vi "Staib EG.vi"(0 "QUIT":refnum<vi>, 1 "Scan in Progress":refnum<vi>, 2 "Set EG":refnum<vi>, 3 "Energy (eV)":refnum<vi>, 4 "Extraction (V)":refnum<vi>, 5 "Filament (V)":refnum<vi>, 6 "EG Computer Control":refnum<vi>, 7 "X1 Alignment (V)":refnum<vi>, 8 "Error":refnum<vi>, 9 "X2 Alignment (V)":refnum<vi>, 11 "Y1 Alignment (V)":refnum<vi>, 13 "Y2 Alignment (V)":refnum<vi>, 14 "Grid (V)":refnum<vi>, 15 "Focus 1 (V)":refnum<vi>, 16 "Focus 2 (V)":refnum<vi>) -> ()   [LabVIEW 2018]
uses:
  <vilib>/DAQmx/write.llb/DAQmx Write (Analog DBL 1Chan 1Samp).vi
  <vilib>/DAQmx/write.llb/DAQmx Write (Digital Bool 1Line 1Point).vi
panel:
  in  "Staib Electron Gun":enum32{"Controls", "Settings"}(tab)
  in  "Lock Focus Knobs":bool
  out "Computer\nControl Enabled?":bool
  in  "Computer\nControl":bool
  in  "Y2 Alignment (V)":dbl(knob) min=-10.0 max=10.0 step=0.001 scale=-10.0..10.0 scale format="%#_3g"
  in  "Y1 Alignment (V)":dbl(knob) min=-10.0 max=10.0 step=0.001 scale=-10.0..10.0 scale format="%#_3g"
  in  "X2 Alignment (V)":dbl(knob) min=-10.0 max=10.0 step=0.001 scale=-10.0..10.0 scale format="%#_3g"
  in  "X1 Alignment (V)":dbl(knob) min=-10.0 max=10.0 step=0.001 scale=-10.0..10.0 scale format="%#_3g"
  in  "Filament (V)":dbl(knob) min=0.0 max=10.0 step=0.001 scale=0.0..5.0 scale format="%#_3g"
  in  "Focus 2 (V)":dbl(knob) min=-0.0 max=0.0 step=0.001 scale=0.0..0.001 scale format="%#_3g"
  in  "Focus 1 (V)":dbl(knob) min=-0.0 max=0.0 step=0.001 scale=0.0..0.001 scale format="%#_3g"
  in  "Extraction (V)":dbl(knob) min=0.0 max=100.0 step=0.001 scale=0.0..100.0 scale format="%#_3g"
  in  "Energy (eV)":dbl(knob) min=0.0 max=100.0 step=0.001 scale=0.0..100.0 scale format="%#_3g"
  in  "Grid (V)":dbl(knob) min=-15.0 max=15.0 step=0.001 scale=-15.0..15.0 scale format="%#_3g"
  out "Feedback Extraction":dbl caption="Ext"
  out "Feedback Filament":dbl caption="Fil"
  out "Feedback Energy":dbl caption="En"
  out "Feedback Grid":dbl caption="G"
  out "Feedback Focus 1":dbl caption="F 1"
  out "Feedback Focus 2":dbl caption="F 2"
  out "Feedback X1 Alignment":dbl caption="X1"
  out "Feedback X2 Alignment":dbl caption="X2"
  out "Feedback Y1 Alignment":dbl caption="Y1"
  out "Feedback Y2 Alignment":dbl caption="Y2"
  out "Focus Max (V)":dbl min=0.0 max=100.0 step=0.001
  out "Focus Min (V)":dbl
  out "Focus Disable":i32
  in  "Minimum Upper Limit of Focus' Scale (V)":dbl=0.001 min=1e-05 max=100.0 step=0.001
  # "Note that there is no feedback from the electron gun's hardware.  Check the controller's LEDs if unsure."
  # "On"
  # "Off"
  # "Software Feedback"
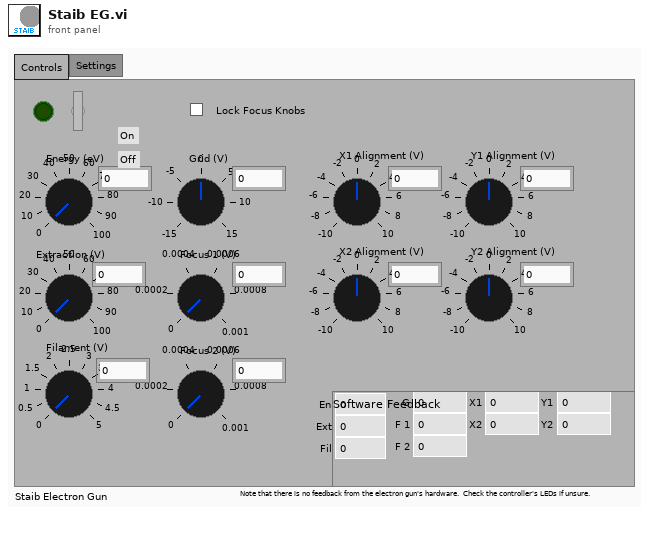
[diagram p1: front panel]
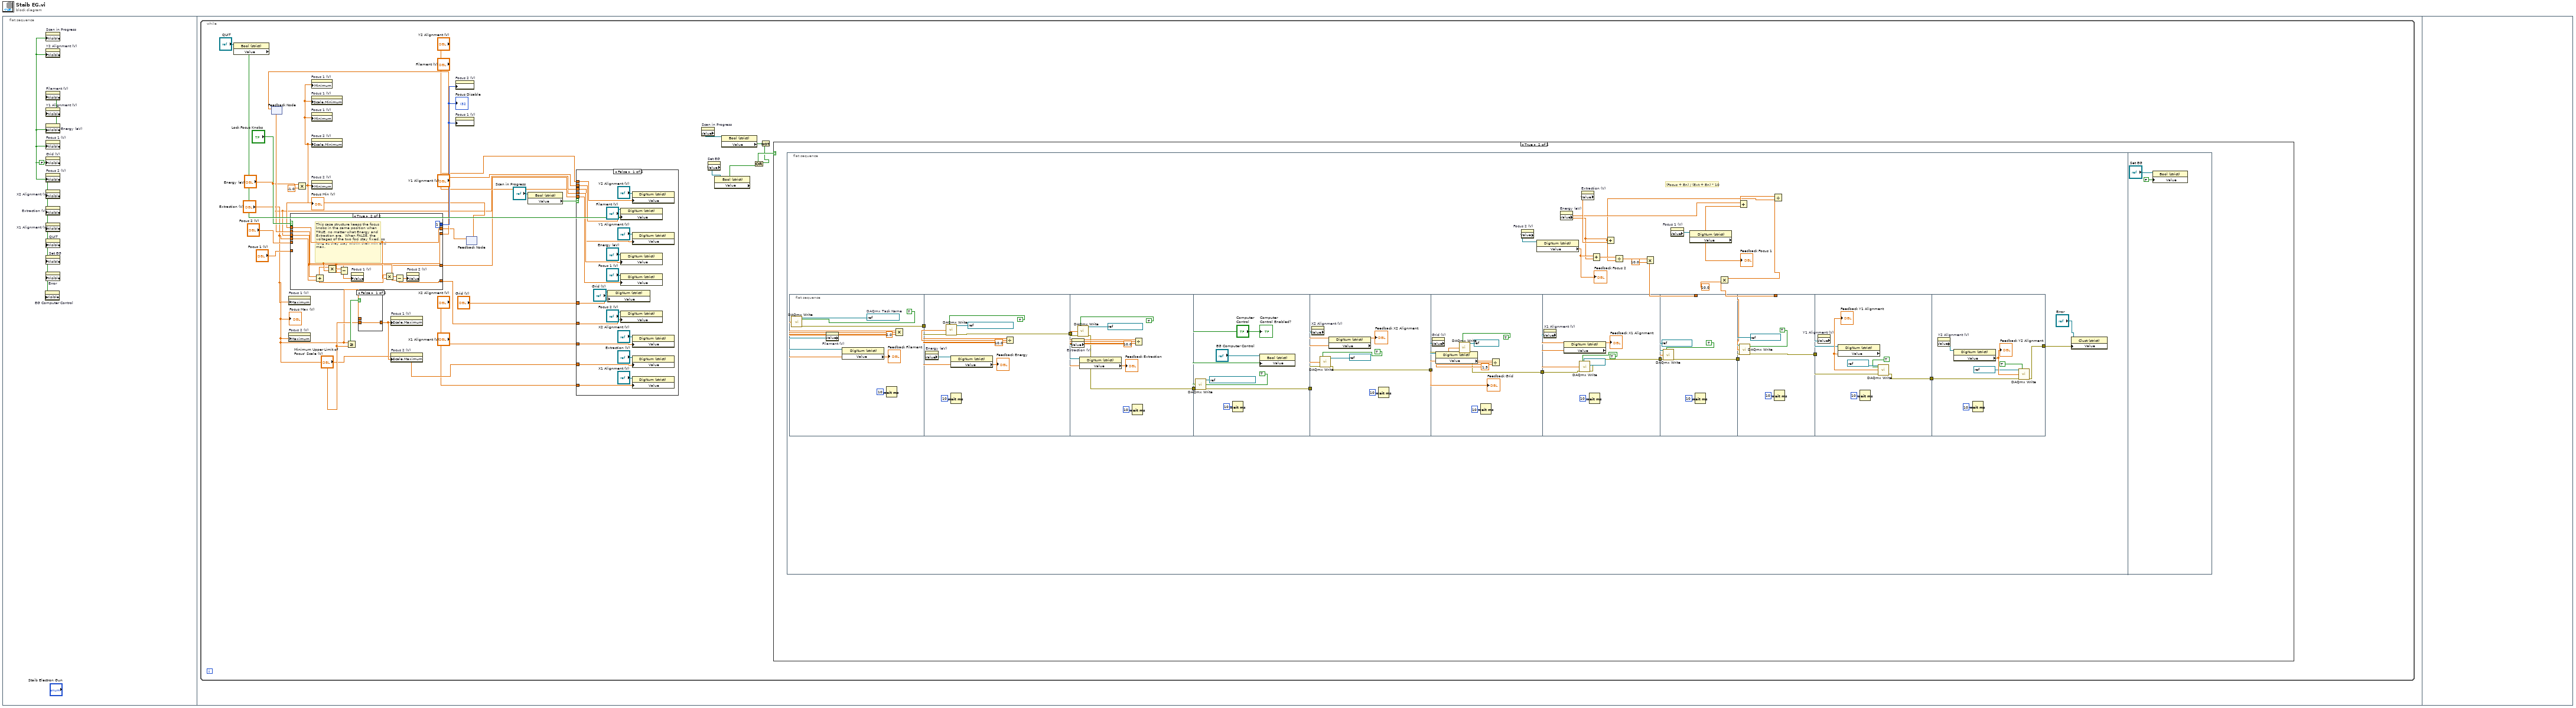
[diagram p0: block diagram]
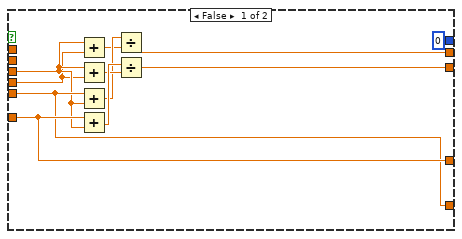
[diagram p5: hidden frame]
diagram:
  n1 = flat-sequence {
    frame #0 {
      w1 = FALSE ("Visible")
      n2 = property on="EG Computer Control" class="LVObjRef (strict)"("Visible"=w1) -> ()  [unwired: 2 in, 2 out]
      n3 = property on="Scan in Progress" class="LVObjRef (strict)"("Visible"=w1) -> ()  [unwired: 2 in, 2 out]
      n4 = property on="Y2 Alignment (V)" class="LVObjRef (strict)"("Visible"=w1) -> ()  [unwired: 2 in, 2 out]
      n5 = property on="Filament (V)" class="LVObjRef (strict)"("Visible"=w1) -> ()  [unwired: 2 in, 2 out]
      n6 = property on="Y1 Alignment (V)" class="LVObjRef (strict)"("Visible"=w1) -> ()  [unwired: 2 in, 2 out]
      n7 = property on="Energy (eV)" class="LVObjRef (strict)"("Visible"=w1) -> ()  [unwired: 2 in, 2 out]
      n8 = property on="Focus 1 (V)" class="LVObjRef (strict)"("Visible"=w1) -> ()  [unwired: 2 in, 2 out]
      n9 = property on="Grid (V)" class="LVObjRef (strict)"("Visible"=w1) -> ()  [unwired: 2 in, 2 out]
      n10 = property on="Focus 2 (V)" class="LVObjRef (strict)"("Visible"=w1) -> ()  [unwired: 2 in, 2 out]
      n11 = property on="X2 Alignment (V)" class="LVObjRef (strict)"("Visible"=w1) -> ()  [unwired: 2 in, 2 out]
      n12 = property on="Extraction (V)" class="LVObjRef (strict)"("Visible"=w1) -> ()  [unwired: 2 in, 2 out]
      n13 = property on="X1 Alignment (V)" class="LVObjRef (strict)"("Visible"=w1) -> ()  [unwired: 2 in, 2 out]
      n14 = property on="QUIT" class="LVObjRef (strict)"("Visible"=w1) -> ()  [unwired: 2 in, 2 out]
      n15 = property on="Set EG" class="LVObjRef (strict)"("Visible"=w1) -> ()  [unwired: 2 in, 2 out]
      n16 = property on="Error" class="LVObjRef (strict)"("Visible"=w1) -> ()  [unwired: 2 in, 2 out]
    }
    frame #1 {
      n17 = while {
        stop <- w33 stop-if-true
        n18 = property class="Bool (strict)"(reference="QUIT") -> ("Value"=w33:bool)  [unwired: 1 in, 2 out]
        n19 = feedback #1() -> (w26:dbl)  [unwired: 1 in]
        n20 = property on="Focus 1 (V)" class="Knob (strict)"("Maximum"="Extraction (V)") -> ()  [unwired: 2 in, 2 out]
        n21 = property on="Focus 2 (V)" class="Knob (strict)"("Maximum"="Extraction (V)") -> ()  [unwired: 2 in, 2 out]
        n22 = Multiply(x="Energy (eV)", y=-1.0) -> (x*y=w21:dbl)
        "Focus Min (V)" <- w21
        n23 = property on="Focus 1 (V)" class="Knob (strict)"("Minimum"=w21) -> ()  [unwired: 2 in, 2 out]
        n24 = property on="Focus 1 (V)" class="Knob (strict)"("Scale.Minimum"=w21) -> ()  [unwired: 2 in, 2 out]
        n25 = property on="Focus 1 (V)" class="Knob (strict)"("Minimum"=w21) -> ()  [unwired: 2 in, 2 out]
        n26 = property on="Focus 2 (V)" class="Knob (strict)"("Scale.Minimum"=w21) -> ()  [unwired: 2 in, 2 out]
        n27 = property on="Focus 2 (V)" class="Knob (strict)"("Minimum"=w21) -> ()  [unwired: 2 in, 2 out]
        n28 = Greater Or Equal?(x="Extraction (V)", y="Minimum Upper Limit of Focus' Scale (V)") -> (x >= y?=w23:bool)
        n29 = case shown="False" w23 {
          tunnel: "Extraction (V)" -> [_ w167]
          tunnel: [w166 w167] -> w22
          tunnel: "Minimum Upper Limit of Focus' Scale (V)" -> [w166 _]
          frame False {
          }
          frame True {
          }
        }
        n30 = property on="Focus 1 (V)" class="Knob (strict)"("Scale.Maximum"=w22) -> ()  [unwired: 2 in, 2 out]
        n31 = property on="Focus 2 (V)" class="Knob (strict)"("Scale.Maximum"=w22) -> ()  [unwired: 2 in, 2 out]
        n32 = feedback #2() -> (w24:dbl)  [unwired: 1 in]
        n33 = case shown="True" "Lock Focus Knobs" {
          tunnel: "Focus 2 (V)" -> [w171 _]
          tunnel: [w171 w179] -> w15
          tunnel: "Focus 1 (V)" -> [w177 _]
          tunnel: [w177 w180] -> w16
          tunnel: [0 1] -> w30
          tunnel: "Energy (eV)" -> [w170 w181]
          tunnel: "Extraction (V)" -> [w169 w187]
          tunnel: [w174 w185] -> w27
          tunnel: [w168 w183] -> w25
          tunnel: w26 -> [_ w185]
          tunnel: w24 -> [_ w183]
          frame False {
            n34 = Add(x=w170, y=w169) -> (x+y=w172:dbl)
            n35 = Add(x=w170, y=w169) -> (x+y=w175:dbl)
            n36 = Add(x=w171, y=w170) -> (x+y=w173:dbl)
            n37 = Add(x=w177, y=w170) -> (x+y=w176:dbl)
            n38 = Divide(x=w173, y=w172) -> (x/y=w168:dbl)
            n39 = Divide(x=w176, y=w175) -> (x/y=w174:dbl)
          }
          frame True {
            # "This case structure keeps the focus knobs in the same position when TRUE, no matter what Energy and Extraction are.  When FALSE, the voltages of the two foci stay fixed, so long as they stay within their min and max."
            n40 = Add(x=w181, y=w187) -> (x+y=w184:dbl)
            n41 = Multiply(x=w184, y=w185) -> (x*y=w186:dbl)
            n42 = Subtract(x=w186, y=w181) -> (x-y=w180:dbl)
            n43 = property on="Focus 1 (V)" class="Knob (strict)"("Value"=w180) -> ()  [unwired: 2 in, 2 out]
            n44 = Multiply(x=w184, y=w183) -> (x*y=w182:dbl)
            n45 = Subtract(x=w182, y=w181) -> (x-y=w179:dbl)
            n46 = property on="Focus 2 (V)" class="Knob (strict)"("Value"=w179) -> ()  [unwired: 2 in, 2 out]
          }
        }
        "Focus Disable" <- w30
        n47 = feedback-in #1(w27) -> ()
        n48 = property on="Focus 2 (V)" class="Knob (strict)"("DisabledEnum"=w30) -> ()  [unwired: 2 in, 2 out]
        n49 = property on="Focus 1 (V)" class="Knob (strict)"("DisabledEnum"=w30) -> ()  [unwired: 2 in, 2 out]
        n50 = feedback-in #2(w25) -> ()
        n51 = property class="Bool (strict)"(reference="Scan in Progress") -> ("Value"=w9:bool)  [unwired: 1 in, 2 out]
        n52 = case shown="False" w9 {
          tunnel: "Energy (eV)" -> [w165 _]
          tunnel: "Extraction (V)" -> [w164 _]
          tunnel: "Filament (V)" -> [w163 _]
          tunnel: "Grid (V)" -> [w162 _]
          tunnel: w16 -> [w161 _]
          tunnel: w15 -> [w160 _]
          tunnel: "X1 Alignment (V)" -> [w159 _]
          tunnel: "X2 Alignment (V)" -> [w158 _]
          tunnel: "Y1 Alignment (V)" -> [w157 _]
          tunnel: "Y2 Alignment (V)" -> [w156 _]
          frame False {
            n53 = property class="DigNum (strict)"(reference="Grid (V)", "Value"=w162) -> ()  [unwired: 1 in, 2 out]
            n54 = property class="DigNum (strict)"(reference="Filament (V)", "Value"=w163) -> ()  [unwired: 1 in, 2 out]
            n55 = property class="DigNum (strict)"(reference="Energy (eV)", "Value"=w165) -> ()  [unwired: 1 in, 2 out]
            n56 = property class="DigNum (strict)"(reference="Focus 1 (V)", "Value"=w161) -> ()  [unwired: 1 in, 2 out]
            n57 = property class="DigNum (strict)"(reference="Focus 2 (V)", "Value"=w160) -> ()  [unwired: 1 in, 2 out]
            n58 = property class="DigNum (strict)"(reference="Y2 Alignment (V)", "Value"=w156) -> ()  [unwired: 1 in, 2 out]
            n59 = property class="DigNum (strict)"(reference="Y1 Alignment (V)", "Value"=w157) -> ()  [unwired: 1 in, 2 out]
            n60 = property class="DigNum (strict)"(reference="X2 Alignment (V)", "Value"=w158) -> ()  [unwired: 1 in, 2 out]
            n61 = property class="DigNum (strict)"(reference="Extraction (V)", "Value"=w164) -> ()  [unwired: 1 in, 2 out]
            n62 = property class="DigNum (strict)"(reference="X1 Alignment (V)", "Value"=w159) -> ()  [unwired: 1 in, 2 out]
          }
          frame True {
          }
        }
        n63 = property on="Scan in Progress" class="LVObjRef (strict)"() -> ("Value"=w8:refnum<vi>)  [unwired: 2 in, 2 out]
        n64 = property on="Set EG" class="LVObjRef (strict)"() -> ("Value"=w6:refnum<vi>)  [unwired: 2 in, 2 out]
        n65 = property class="Bool (strict)"(reference=w6) -> ("Value"=w5:bool)  [unwired: 1 in, 2 out]
        n66 = property class="Bool (strict)"(reference=w8) -> ("Value"=w7:bool)  [unwired: 1 in, 2 out]
        n67 = Not(x=w7) -> (.not. x?=w3:bool)
        n68 = Or(x=w3, y=w5) -> (x .or. y?=w4:bool)
        n69 = case shown="True" w4 {
          frame False {
          }
          frame True {
            n70 = flat-sequence {
              frame #0 {
                # "(Focus + En) / (Ext + En) * 10"
                n71 = flat-sequence {
                  tunnel: [w63] -> w47
                  tunnel: w47 -> [w72]
                  tunnel: [w71] -> w46
                  tunnel: w46 -> [w81]
                  tunnel: [w80] -> w45
                  tunnel: w45 -> [w90]
                  tunnel: [w89] -> w44
                  tunnel: w44 -> [w97]
                  tunnel: [w96] -> w43
                  tunnel: w43 -> [w104]
                  tunnel: [w103] -> w42
                  tunnel: w42 -> [w113]
                  tunnel: [w112] -> w40
                  tunnel: w41 -> [w122]
                  tunnel: w40 -> [w121]
                  tunnel: [w119] -> w39
                  tunnel: w39 -> [w126]
                  tunnel: w38 -> [w127]
                  tunnel: [w125] -> w37
                  tunnel: w37 -> [w132]
                  tunnel: [w131] -> w36
                  tunnel: w36 -> [w139]
                  tunnel: [w138] -> w35
                  frame #0 {
                    w65 = refnum<k21> "Filament out"  # DAQmx Task Name
                    n72 = property on="Filament (V)" class="LVObjRef (strict)"() -> ("Value"=w68:refnum<vi>)  [unwired: 2 in, 2 out]
                    n73 = property class="DigNum (strict)"(reference=w68) -> ("Value"=w69:dbl)  [unwired: 1 in, 2 out]
                    "Feedback Filament" <- w69
                    n74 = Wait (ms)(milliseconds to wait=u32 10) -> ()  [unwired: 1 out]
                    n75 = Multiply(x=w69, y=2.0) -> (x*y=w67:dbl)
                    n76 = call-poly <vilib>:"DAQmx Write.vi"("task/channels in"=w65, "auto start"=TRUE, "data"=w67) -> ("error out"=w63:errorcluster)  [unwired: 10 in, 2 out]
                  }
                  frame #1 {
                    n77 = property on="Energy (eV)" class="LVObjRef (strict)"() -> ("Value"=w77:refnum<vi>)  [unwired: 2 in, 2 out]
                    n78 = property class="DigNum (strict)"(reference=w77) -> ("Value"=w78:dbl)  [unwired: 1 in, 2 out]
                    "Feedback Energy" <- w78
                    n79 = Wait (ms)(milliseconds to wait=u32 10) -> ()  [unwired: 1 out]
                    n80 = Divide(x=w78, y=10.0) -> (x/y=w76:dbl)
                    n81 = call-poly <vilib>:"DAQmx Write.vi"("task/channels in"=refnum<k21> "Electron Energy Out", "auto start"=TRUE, "data"=w76, "error in"=w72) -> ("error out"=w71:errorcluster)  [unwired: 9 in, 2 out]
                  }
                  frame #2 {
                    n82 = property on="Extraction (V)" class="LVObjRef (strict)"() -> ("Value"=w86:refnum<vi>)  [unwired: 2 in, 2 out]
                    n83 = property class="DigNum (strict)"(reference=w86) -> ("Value"=w87:dbl)  [unwired: 1 in, 2 out]
                    "Feedback Extraction" <- w87
                    n84 = Wait (ms)(milliseconds to wait=u32 10) -> ()  [unwired: 1 out]
                    n85 = Divide(x=w87, y=10.0) -> (x/y=w85:dbl)
                    n86 = call-poly <vilib>:"DAQmx Write.vi"("task/channels in"=refnum<k21> "Extraction out", "auto start"=TRUE, "data"=w85, "error in"=w81) -> ("error out"=w80:errorcluster)  [unwired: 9 in, 2 out]
                  }
                  frame #3 {
                    n87 = call-poly <vilib>:"DAQmx Write.vi"("task/channels in"=refnum<k21> "ElectronCPUControl", "auto start"=TRUE, "data"="Computer\nControl", "error in"=w90) -> ("error out"=w89:errorcluster)  [unwired: 9 in, 2 out]
                    n88 = Wait (ms)(milliseconds to wait=u32 10) -> ()  [unwired: 1 out]
                    n89 = property class="Bool (strict)"(reference="EG Computer Control", "Value"="Computer\nControl") -> ()  [unwired: 1 in, 2 out]
                    "Computer\nControl Enabled?" <- "Computer\nControl"
                  }
                  frame #4 {
                    n90 = property on="X2 Alignment (V)" class="LVObjRef (strict)"() -> ("Value"=w100:refnum<vi>)  [unwired: 2 in, 2 out]
                    n91 = property class="DigNum (strict)"(reference=w100) -> ("Value"=w101:dbl)  [unwired: 1 in, 2 out]
                    "Feedback X2 Alignment" <- w101
                    n92 = call-poly <vilib>:"DAQmx Write.vi"("task/channels in"=refnum<k21> "X2 out", "auto start"=TRUE, "data"=w101, "error in"=w97) -> ("error out"=w96:errorcluster)  [unwired: 9 in, 2 out]
                    n93 = Wait (ms)(milliseconds to wait=u32 10) -> ()  [unwired: 1 out]
                  }
                  frame #5 {
                    n94 = property on="Grid (V)" class="LVObjRef (strict)"() -> ("Value"=w109:refnum<vi>)  [unwired: 2 in, 2 out]
                    n95 = property class="DigNum (strict)"(reference=w109) -> ("Value"=w110:dbl)  [unwired: 1 in, 2 out]
                    "Feedback Grid" <- w110
                    n96 = Wait (ms)(milliseconds to wait=u32 10) -> ()  [unwired: 1 out]
                    n97 = Divide(x=w110, y=1.5) -> (x/y=w108:dbl)
                    n98 = call-poly <vilib>:"DAQmx Write.vi"("task/channels in"=refnum<k21> "Grid Out", "auto start"=TRUE, "data"=w108, "error in"=w104) -> ("error out"=w103:errorcluster)  [unwired: 9 in, 2 out]
                  }
                  frame #6 {
                    n99 = property on="X1 Alignment (V)" class="LVObjRef (strict)"() -> ("Value"=w116:refnum<vi>)  [unwired: 2 in, 2 out]
                    n100 = property class="DigNum (strict)"(reference=w116) -> ("Value"=w117:dbl)  [unwired: 1 in, 2 out]
                    "Feedback X1 Alignment" <- w117
                    n101 = call-poly <vilib>:"DAQmx Write.vi"("task/channels in"=refnum<k21> "X1 out", "auto start"=TRUE, "data"=w117, "error in"=w113) -> ("error out"=w112:errorcluster)  [unwired: 9 in, 2 out]
                    n102 = Wait (ms)(milliseconds to wait=u32 10) -> ()  [unwired: 1 out]
                  }
                  frame #7 {
                    n103 = call-poly <vilib>:"DAQmx Write.vi"("task/channels in"=refnum<k21> "Focus 2 out", "auto start"=TRUE, "data"=w122, "error in"=w121) -> ("error out"=w119:errorcluster)  [unwired: 9 in, 2 out]
                    n104 = Wait (ms)(milliseconds to wait=u32 10) -> ()  [unwired: 1 out]
                  }
                  frame #8 {
                    n105 = call-poly <vilib>:"DAQmx Write.vi"("task/channels in"=refnum<k21> "Focus 1 out", "auto start"=TRUE, "data"=w127, "error in"=w126) -> ("error out"=w125:errorcluster)  [unwired: 9 in, 2 out]
                    n106 = Wait (ms)(milliseconds to wait=u32 10) -> ()  [unwired: 1 out]
                  }
                  frame #9 {
                    n107 = property on="Y1 Alignment (V)" class="LVObjRef (strict)"() -> ("Value"=w135:refnum<vi>)  [unwired: 2 in, 2 out]
                    n108 = property class="DigNum (strict)"(reference=w135) -> ("Value"=w136:dbl)  [unwired: 1 in, 2 out]
                    "Feedback Y1 Alignment" <- w136
                    n109 = Wait (ms)(milliseconds to wait=u32 10) -> ()  [unwired: 1 out]
                    n110 = call-poly <vilib>:"DAQmx Write.vi"("task/channels in"=refnum<k21> "Y1 out", "auto start"=TRUE, "data"=w136, "error in"=w132) -> ("error out"=w131:errorcluster)  [unwired: 9 in, 2 out]
                  }
                  frame #10 {
                    n111 = property on="Y2 Alignment (V)" class="LVObjRef (strict)"() -> ("Value"=w142:refnum<vi>)  [unwired: 2 in, 2 out]
                    n112 = property class="DigNum (strict)"(reference=w142) -> ("Value"=w143:dbl)  [unwired: 1 in, 2 out]
                    "Feedback Y2 Alignment" <- w143
                    n113 = Wait (ms)(milliseconds to wait=u32 10) -> ()  [unwired: 1 out]
                    n114 = call-poly <vilib>:"DAQmx Write.vi"("task/channels in"=refnum<k21> "Y2 out", "auto start"=TRUE, "data"=w143, "error in"=w139) -> ("error out"=w138:errorcluster)  [unwired: 9 in, 2 out]
                  }
                }
                n115 = property on="Focus 2 (V)" class="LVObjRef (strict)"() -> ("Value"=w60:refnum<vi>)  [unwired: 2 in, 2 out]
                n116 = property class="DigNum (strict)"(reference=w60) -> ("Value"=w56:dbl)  [unwired: 1 in, 2 out]
                "Feedback Focus 2" <- w56
                n117 = property on="Energy (eV)" class="Knob (strict)"() -> ("Value"=w51:dbl)  [unwired: 2 in, 2 out]
                n118 = property on="Extraction (V)" class="Knob (strict)"() -> ("Value"=w57:dbl)  [unwired: 2 in, 2 out]
                n119 = Add(x=w56, y=w51) -> (x+y=w55:dbl)
                n120 = Add(x=w51, y=w57) -> (x+y=w49:dbl)
                n121 = Divide(x=w55, y=w49) -> (x/y=w54:dbl)
                n122 = Multiply(x=w54, y=10.0) -> (x*y=w41:dbl)
                n123 = property on="Focus 1 (V)" class="LVObjRef (strict)"() -> ("Value"=w59:refnum<vi>)  [unwired: 2 in, 2 out]
                n124 = property class="DigNum (strict)"(reference=w59) -> ("Value"=w52:dbl)  [unwired: 1 in, 2 out]
                "Feedback Focus 1" <- w52
                n125 = Add(x=w51, y=w52) -> (x+y=w50:dbl)
                n126 = Divide(x=w50, y=w49) -> (x/y=w48:dbl)
                n127 = Multiply(x=w48, y=10.0) -> (x*y=w38:dbl)
                n128 = property class="Clust (strict)"(reference="Error", "Value"=w35) -> ()  [unwired: 1 in, 2 out]
              }
              frame #1 {
                n129 = property class="Bool (strict)"(reference="Set EG", "Value"=FALSE) -> ()  [unwired: 1 in, 2 out]
              }
            }
          }
        }
        "Focus Max (V)" <- "Extraction (V)"
      }
    }
    frame #2 {
    }
  }
